vi "Identify Worst Tone at Target Pout per Tone.vi"(7 "Target Pout Per Tone (dBm)":dbl, 9 "OIP3 Upper":dbl[](array[numeric]), 10 "OIP3 Lower":dbl[](array[numeric]), 11 "Pout per Tone (dBm)":dbl[](array[numeric])) -> (3 "Worst TOI lower?":bool)   [LabVIEW 2023]
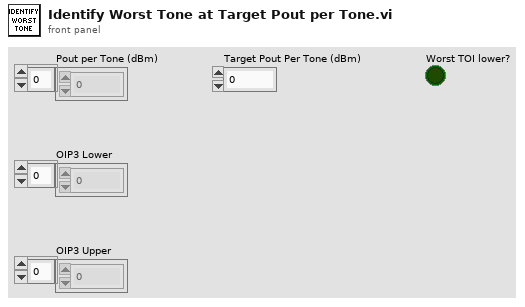
[diagram p1: front panel]
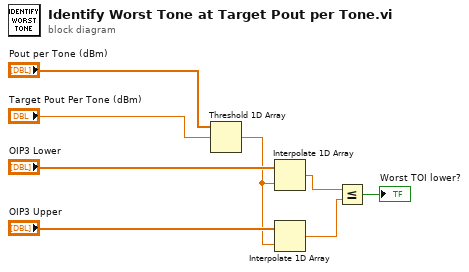
[diagram p0: block diagram]
diagram:
  n1 = Threshold 1D Array(2:"Target Pout Per Tone (dBm)", 3:"Pout per Tone (dBm)") -> (0:w4:dbl)  [unwired: 1 in]
  n2 = Interpolate 1D Array(1:w4, 2:"OIP3 Lower") -> (0:w3:dbl)
  n3 = Interpolate 1D Array(1:w4, 2:"OIP3 Upper") -> (0:w2:dbl)
  n4 = Less Or Equal?(x=w3, y=w2) -> (x <= y?=→"Worst TOI lower?":bool)
